vi "Parse.vi"(0 "Command Array":string[](array[string])) -> (1 "Parameters":string[](array[string]), 2 "Command":string)   [LabVIEW 2015]
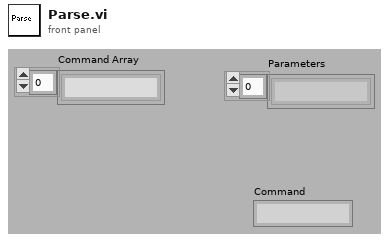
[diagram p1: front panel]
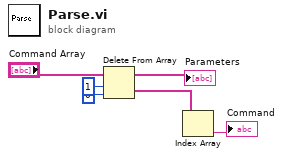
[diagram p0: block diagram]
diagram:
  n1 = Delete From Array(array="Command Array", length=1, index=0) -> (deleted portion=w2:string[], array with subset deleted=→"Parameters":string[])
  n2 = Index Array(array=w2) -> (element=→"Command":string)  [unwired: 1 in]
